vi "LeadScrewFGV.vi"(7 "Function":enum16{"init LC", "Set LC (cm)", "read LC"}(ring), 8 "error in (no error)":errorcluster, 10 "Set LC (cm)":dbl, 11 "miniOut in":T1) -> (0 "error out":errorcluster, 2 "LC position now (cm)":dbl, 3 "miniOut out":T1)   [LabVIEW 2019]
uses:
  <vilib>/ReMiSYS/ReMiSYS_myRIO-mini/SubVI/SYS/miniRef.ctl
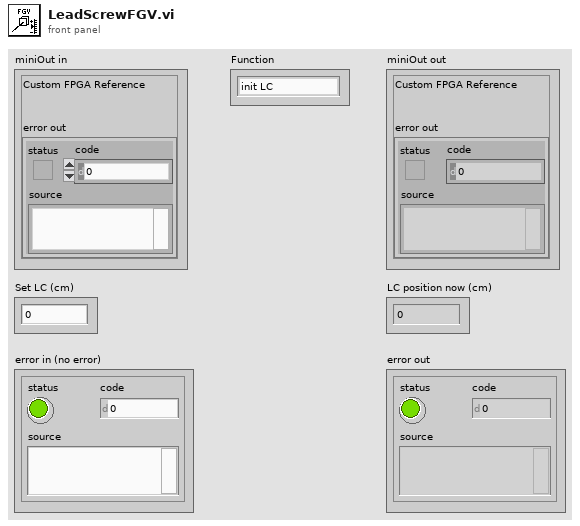
[diagram p1: front panel]
types:
  T1 = typedef "miniRef.ctl" = cluster{"Custom FPGA Reference":refnum<k20>, "error out":errorcluster}
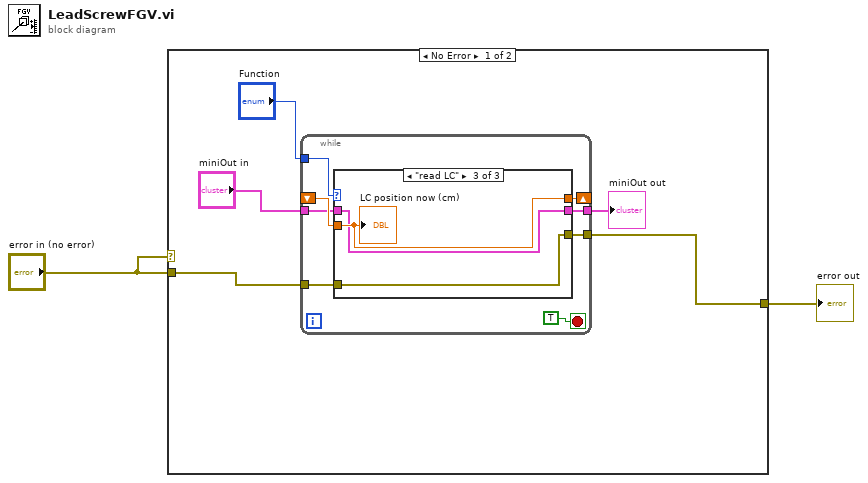
[diagram p0: block diagram]
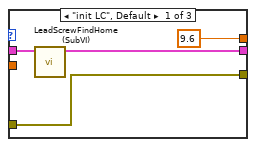
[diagram p2: hidden frame]
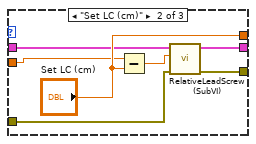
[diagram p3: hidden frame]
diagram:
  n1 = case shown="No Error" "error in (no error)" {
    tunnel: "error in (no error)" -> [w4 w30]
    tunnel: [w3 w30] -> w2
    frame No Error {
      n2 = while {
        tunnel: "Function" -> [w14]
        shift-right: [w13] -> _
        shift-left: _ -> [w12]
        tunnel: "miniOut in" -> [w11]
        tunnel: [w10] -> w5
        tunnel: w4 -> [w9]
        tunnel: [w8] -> w3
        stop <- TRUE stop-if-true
        n3 = case shown="\"read LC\"" w14 {
          tunnel: [9.6 ("Distance (cm)") "Set LC (cm)" w29] -> w13
          tunnel: w12 -> [_ w25 w29]
          tunnel: w11 -> [w18 w23 w28]
          tunnel: [w17 w22 w28] -> w10
          tunnel: w9 -> [w16 w21 w27]
          tunnel: [w16 w20 w27] -> w8
          frame "init LC", Default {
            n4 = call "LeadScrewFindHome (SubVI).vi"("miniOut in"=w18) -> ("miniOut out"=w17:T1)  [unwired: 7 in, 3 out]
          }
          frame "Set LC (cm)" {
            n5 = Subtract(x=w25, y="Set LC (cm)") -> (x-y=w24:dbl)
            n6 = call "RelativeLeadScrew (SubVI).vi"("error in (no error)"=w21, "Distance (cm)"=w24, "miniOut in"=w23) -> ("error out"=w20:errorcluster, "miniOut out"=w22:T1)  [unwired: 5 in, 2 out]
          }
          frame "read LC" {
            "LC position now (cm)" <- w29
          }
        }
      }
      "miniOut out" <- w5
    }
    frame Error {
    }
  }
  "error out" <- w2
